vi "BUILD_install upload.vi"() -> ()   [LabVIEW 2013]
panel:
  out "error out":errorcluster
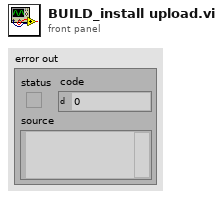
[diagram p1: front panel]
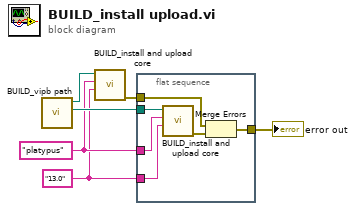
[diagram p0: block diagram]
diagram:
  w2 = "platypus" ("Repository Name")
  w1 = "13.0" ("LabVIEW Version")
  n1 = call "BUILD_vipb path.vi"() -> ("2"=w3:path, "appended path"=w5:path)  [unwired: 10 in]
  n2 = call "BUILD_install and upload core.vi"("LabVIEW Version"=w1, "Repository Name"=w2, "appended path"=w5) -> ("error out"=w6:errorcluster)  [unwired: 8 in]
  n3 = flat-sequence {
    tunnel: w6 -> [w12]
    tunnel: [w11] -> w4
    tunnel: w3 -> [w9]
    tunnel: w2 -> [w8]
    tunnel: w1 -> [w7]
    frame #0 {
      n4 = call "BUILD_install and upload core.vi"("LabVIEW Version"=w7, "Repository Name"=w8, "appended path"=w9) -> ("error out"=w10:errorcluster)  [unwired: 8 in]
      n5 = Merge Errors(w12, w10) -> (w11:errorcluster)
    }
  }
  "error out" <- w4
